vi "New Results (to override).vi"(7 "Image Nr.":i32, 8 "error in (no error)":errorcluster, 9 "Results In":refnum<class "Analyze Results Base.lvclass">[](array[class]), 10 "Parameters":refnum<class "Analyze Parameter Base.lvclass">[](array[class]), 11 "Launch IMAQ Display in":refnum<class "HIJ Vision File Viewer App.lvclass">) -> (0 "error out":errorcluster, 3 "Launch IMAQ Display out":refnum<class "HIJ Vision File Viewer App.lvclass">)   [LabVIEW 2014, in "HIJ Vision File Viewer App.lvlib" / "HIJ Vision File Viewer App.lvclass"]
uses:
  HIJ Vision File Viewer App.lvclass
  HIJ Vision Application/HIJ Vision Application/HIJ Vision Application.lvclass
  Analyze/Results and Overlays/Results Base/Analyze Results Base.lvclass
  Analyze/Analyze Parameter/Analyze Parameter Base/Analyze Parameter Base.lvclass
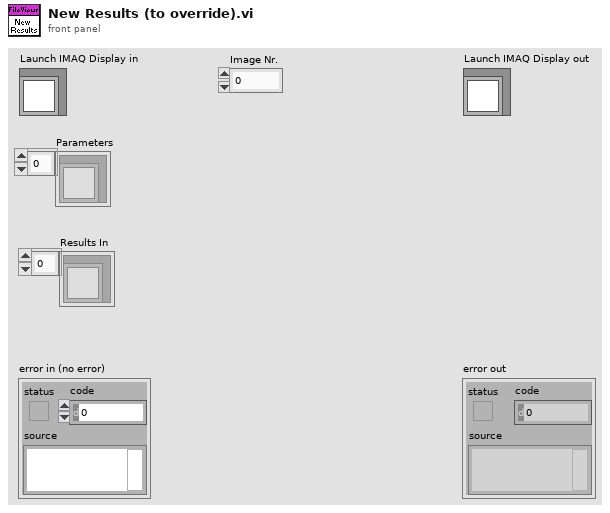
[diagram p1: front panel]
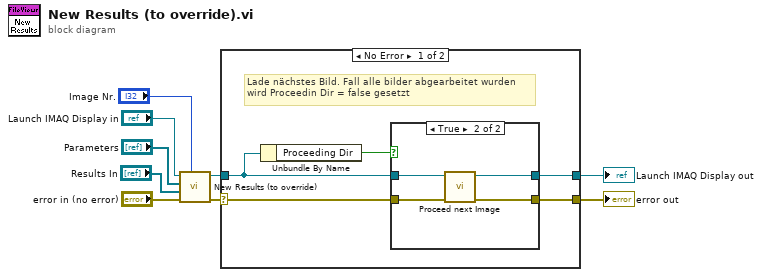
[diagram p0: block diagram]
diagram:
  n1 = call-parent "New Results (to override).vi"("Image Nr."="Image Nr.", "error in (no error)"="error in (no error)", "Results In"="Results In", "Parameters"="Parameters", "Launch IMAQ Display in"="Launch IMAQ Display in") -> ("error out"=w2:errorcluster, "Launch IMAQ Display out"=w4:refnum<class "HIJ Vision File Viewer App.lvclass">)  [unwired: 5 in]
  n2 = case shown="No Error" w2 {
    selector: w2 -> [w10 w22]
    tunnel: [w14 w21] -> w5
    tunnel: w4 -> [w13 w21]
    tunnel: [w12 w22] -> w3
    frame No Error {
      # "Lade nächstes Bild. Fall alle bilder abgearbeitet wurden\nwird Proceedin Dir = false gesetzt"
      n3 = Unbundle By Name(w13) -> ("Proceeding Dir"=w11:bool)
      n4 = case shown="True" w11 {
        tunnel: [w16 w20] -> w14
        tunnel: w13 -> [w16 w19]
        tunnel: w10 -> [w15 w18]
        tunnel: [w15 w17] -> w12
        frame False {
        }
        frame True {
          n5 = call-dynamic "Proceed next Image.vi"("error in (no error)"=w18, "Launch File Viewer in"=w19) -> ("error out"=w17:errorcluster, "Launch File Viewer out"=w20:refnum<class "HIJ Vision File Viewer App.lvclass">)  [unwired: 8 in]
        }
      }
    }
    frame Error {
    }
  }
  "error out" <- w3
  "Launch IMAQ Display out" <- w5
